vi "Аккумулятор.vi"(1 "Reset":bool, 2 "C":bool, 3 "d":T1) -> (0 "output cluster":T2)   [LabVIEW 2012]
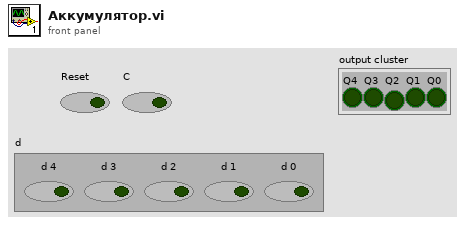
[diagram p1: front panel]
types:
  T1 = cluster{"d 4":bool, "d 3":bool, "d 2 ":bool, "d 1":bool, "d 0":bool}
  T2 = cluster{"Q4":bool, "Q3":bool, "Q2":bool, "Q1":bool, "Q0":bool}
  T3 = cluster{"q":bool, "q":bool, "q":bool, "q":bool, "q":bool}
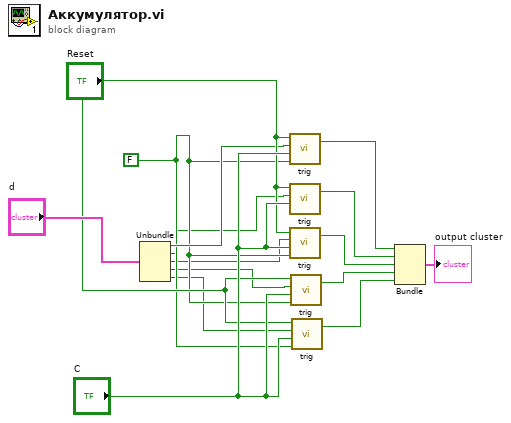
[diagram p0: block diagram]
diagram:
  w5 = FALSE
  n1 = Unbundle("d") -> ("d 4"=w6:bool, "d 3"=w4:bool, "d 2"=w3:bool, "d 1"=w2:bool, "d 0"=w1:bool)
  n2 = call "trig.vi"("s"=w5, "c"="C", "d"=w6, "r"="Reset") -> ("q"=w10:bool)  [unwired: 1 out]
  n3 = call "trig.vi"("c"="C", "d"=w4, "r"="Reset") -> ("q"=w11:bool)  [unwired: 1 in, 1 out]
  n4 = call "trig.vi"("s"=w5, "c"="C", "d"=w3, "r"="Reset") -> ("q"=w12:bool)  [unwired: 1 out]
  n5 = call "trig.vi"("s"=w5, "c"="C", "d"=w2, "r"="Reset") -> ("q"=w13:bool)  [unwired: 1 out]
  n6 = call "trig.vi"("s"=w5, "c"="C", "d"=w1, "r"="Reset") -> ("q"=w14:bool)  [unwired: 1 out]
  n7 = Bundle("q"=w10, "q"=w11, "q"=w12, "q"=w13, "q"=w14) -> (→"output cluster":T3)  [unwired: 1 in]
